vi "FIB zoom image draw milling.vi"(0 "Milling Z voltage":dbl, 3 "Milling para":T1={"X resolution"=4096, "Z resolution"=125001, "X offset (um)"=0.0, "Z offset (um)"=0.0, "X center (um)"=0.0, "Z center (um)"=0.0, "X size (um)"=250.0, "Z size (um)"=250.0, "UL-Ang"=90.0, "UR-Ang"=90.0, "Line milling time (s)"=5.0, "Z-step (nm)"=2.0, "Lines auto pause"=1, "Auto pause"=FALSE, "Mill from Bottom"=FALSE, "FIB FOV (um)"=500.0, "Auto Profile"=FALSE, "Mill start from Last"=FALSE, "FIB PID on"=FALSE, "FIB PID reset"=TRUE, "FIB PID measured"=0, "FIB PID target"=0.0, "FIB PID target slope"=0.0, "FIB PID P"=0.001, "FIB PID I"=0.01, "FIB PID D"=0.0, "Emission (uA)"=1.36, "Suppressor (V)"=50.0, "Auto reheat"=FALSE} caption="Milling Parameters" {"Suppressor (V)" step=0.1 format="%.1g"; "Emission (uA)" step=0.1 format="%.2g"; "FIB PID measured" items=["Spec.", "B.D. 1", "B.D. 2", "Mill", "Spec. +"]; "FIB PID target slope" min=-1 max=1 step=0.1; "UR-Ang" format="%.2f"; "UL-Ang" format="%.2f"; "Z offset (um)" step=0.02 format="%.3g"; "X offset (um)" step=1 format="%.3g"; "FIB FOV (um)" format="%.3g"; "Line milling time (s)" format="%.1f"; "Z center (um)" format="%#.3g"; "X center (um)" format="%#.3g"}, 4 "Z offset pre (um)":sgl, 6 "X offset pre (um)":sgl, 7 "FIB Zoom Parameters":T2={"X resolution"=500, "Z resolution"=50, "X center"=0.0, "Z center"=0.0, "X size (V)"=0.0, "Z size (V)"=0.0, "Frame line rampdown ratio"=-0.1, "Scan rate (Hz)"=2000000, "Oversampling"=2} {"Frame line rampdown ratio" min=-1.0 max=1.0 step=0.05 format="%.2g"; "Scan rate (Hz)" max=4000000 format="%#.6p"}, 8 "FIB Options":T3={"Scan mode"=0, "Flip x"=TRUE, "Flip z"=TRUE, "Det"=0} {"Scan mode" items=["Raster", "Serpentine"]; "Det" items=["Detector A", "Detector B"]}, 9 "FIB Scan Parameters":T2={"X resolution"=512, "Z resolution"=512, "X center"=0.0, "Z center"=0.0, "X size (V)"=10.0, "Z size (V)"=10.0, "Frame line rampdown ratio"=-0.1, "Scan rate (Hz)"=2000000, "Oversampling"=2} {"Z size (V)" min=0.0 max=20.0; "X size (V)" min=0.0 max=20.0; "Frame line rampdown ratio" min=-1.0 max=1.0 step=0.05 format="%.2g"; "Scan rate (Hz)" max=4000000 format="%#.6p"; "Z resolution" max=2048; "X resolution" max=2048}, 10 "Pre image":bool, 11 "Image reference":refnum<vi>) -> ()   [LabVIEW 2018]
panel:
  # "Direction"
  # "Start\nfrom"
  # "<"
  # "Flip"
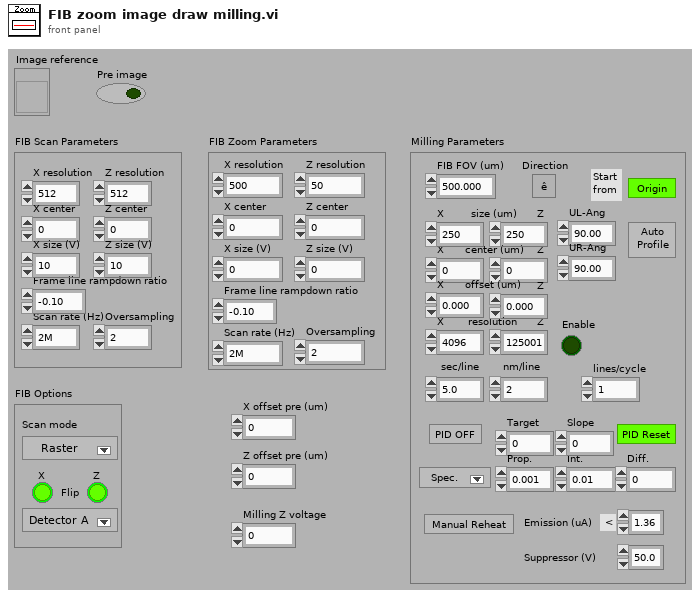
[diagram p1: front panel]
types:
  T1 = cluster{"X resolution":u32, "Z resolution":u32, "X offset (um)":sgl, "Z offset (um)":sgl, "X center (um)":sgl, "Z center (um)":sgl, "X size (um)":sgl, "Z size (um)":sgl, "UL-Ang":sgl, "UR-Ang":sgl, "Line milling time (s)":sgl, "Z-step (nm)":dbl, "Lines auto pause":u16, "Auto pause":bool, "Mill from Bottom":bool, "FIB FOV (um)":sgl, "Auto Profile":bool, "Mill start from Last":bool, "FIB PID on":bool, "FIB PID reset":bool, "FIB PID measured":u8, "FIB PID target":sgl, "FIB PID target slope":sgl, "FIB PID P":sgl, "FIB PID I":sgl, "FIB PID D":sgl, "Emission (uA)":dbl, "Suppressor (V)":sgl, "Auto reheat":bool}
  T2 = cluster{"X resolution":u32, "Z resolution":u32, "X center":dbl, "Z center":dbl, "X size (V)":dbl, "Z size (V)":dbl, "Frame line rampdown ratio":dbl, "Scan rate (Hz)":u32, "Oversampling":u16}
  T3 = cluster{"Scan mode":u16, "Flip x":bool, "Flip z":bool, "Det":u16}
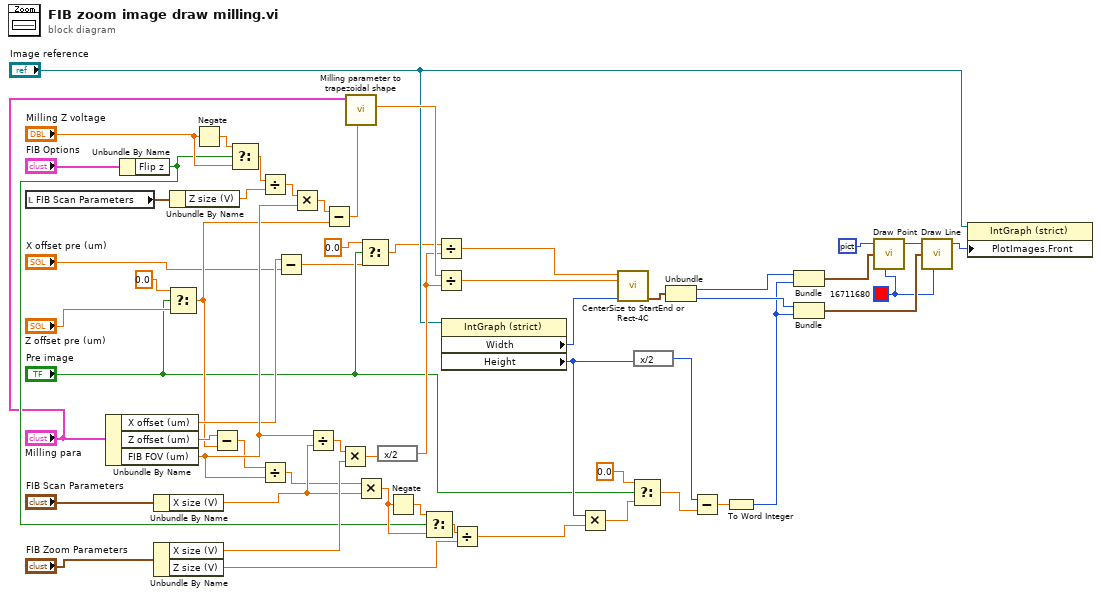
[diagram p0: block diagram]
diagram:
  w27 = u32 16711680 ("color(black)")
  n1 = local read "FIB Scan Parameters"() -> (w49:T2)
  n2 = Unbundle By Name("Milling para") -> ("X offset (um)"=w46:sgl, "Z offset (um)"=w48:sgl, "FIB FOV (um)"=w54:sgl)
  n3 = Unbundle By Name("FIB Options") -> ("Flip z"=w14:bool)
  n4 = Unbundle By Name("FIB Scan Parameters") -> ("X size (V)"=w40:dbl)
  n5 = Unbundle By Name("FIB Zoom Parameters") -> ("X size (V)"=w42:dbl, "Z size (V)"=w22:dbl)
  n6 = Select(t=0.0, s="Pre image", f="Z offset pre (um)") -> (s? t:f=w8:dbl)
  n7 = Unbundle By Name(w49) -> ("Z size (V)"=w50:dbl)
  n8 = Negate(x="Milling Z voltage") -> (-x=w56:dbl)
  n9 = Subtract(x=w48, y=w8) -> (x-y=w47:dbl)
  n10 = Select(t=w56, s=w14, f="Milling Z voltage") -> (s? t:f=w57:dbl)
  n11 = Divide(x=w57, y=w50) -> (x/y=w52:dbl)
  n12 = Divide(x=w47, y=w54) -> (x/y=w33:dbl)
  n13 = Subtract(x=w46, y="X offset pre (um)") -> (x-y=w3:sgl)
  n14 = Multiply(x=w52, y=w54) -> (x*y=w51:dbl)
  n15 = Divide(x=w54, y=w40) -> (x/y=w41:dbl)
  n16 = Subtract(x=w51, y=w8) -> (x-y=w53:dbl)
  n17 = Multiply(x=w41, y=w42) -> (x*y=w43:dbl)
  n18 = call "Milling parameter to trapezoidal shape.vi"("Y location (um)"=w53, "Milling para"="Milling para") -> ("X size (um) @ Y"=w55:dbl)  [unwired: 5 in, 4 out]
  n19 = Multiply(x=w33, y=w40) -> (x*y=w34:dbl)
  n20 = Select(t=0.0, s="Pre image", f=w3) -> (s? t:f=w2:dbl)
  n21 = expression code="x/2"(w43) -> (w44:dbl)
  n22 = Negate(x=w34) -> (-x=w31:dbl)
  n23 = Select(t=w31, s=w14, f=w34) -> (s? t:f=w32:dbl)
  n24 = Divide(x=w2, y=w44) -> (x/y=w35:dbl)
  n25 = Divide(x=w55, y=w44) -> (x/y=w36:dbl)
  n26 = property on="Property Node" class="IntGraph (strict)"(reference="Image reference") -> ("Width"=w45:u32, "Height"=w19:u32)  [unwired: 1 in, 2 out]
  n27 = Divide(x=w32, y=w22) -> (x/y=w23:dbl)
  n28 = Multiply(x=w19, y=w23) -> (x*y=w13:dbl)
  n29 = call "CenterSize to StartEnd or Rect-4C.vi"("Resolution"=w45, "Size"=w36, "Center"=w35) -> ("Rect-4C"=w37:cluster{"left":i16, "right":i16})  [unwired: 2 in, 2 out]
  n30 = Select(t=0.0, s="Pre image", f=w13) -> (s? t:f=w12:dbl)
  n31 = expression code="x/2"(w19) -> (w24:u32)
  n32 = Unbundle(w37) -> ("left"=w38:i16, "right"=w39:i16)
  n33 = Subtract(x=w24, y=w12) -> (x-y=w25:dbl)
  n34 = To Word Integer(number=w25) -> (16bit integer=w28:i16)
  n35 = Bundle("left"=w38, w28) -> (w26:cluster{"left":i16, i16})  [unwired: 1 in]
  n36 = Bundle("right"=w39, w28) -> (w29:cluster{"right":i16, i16})  [unwired: 1 in]
  n37 = call <vilib>:"Draw Point.vi"("picture"=picture data[5B], "point(x,y)"=w26, "color(black)"=w27) -> ("new picture"=w21:picture)  [unwired: 6 in]
  n38 = call <vilib>:"Draw Line.vi"("picture"=w21, "end point"=w29, "color(black)"=w27) -> ("new picture"=w30:picture)  [unwired: 6 in]
  n39 = property on="Property Node" class="IntGraph (strict)"(reference="Image reference", "PlotImages.Front"=w30) -> ()  [unwired: 1 in, 2 out]
